vi "BTB Data Parser.vi"(8 "error in (no error)":errorcluster, 10 "RDS Serial Frame in":refnum<class "RDS Serial Frame.lvclass">, 11 "Battery Instrument in":refnum<class "Battery Instrument.lvclass">) -> (0 "error out":errorcluster, 2 "Battery Message out":refnum<class "Battery Message.lvclass">, 3 "Battery Instrument out":refnum<class "Battery Instrument.lvclass">)   [LabVIEW 2015, in "Battery Instrument.lvlib" / "Battery Instrument.lvclass"]
uses:
  Battery Instrument.lvclass
  Libraries/RDS Serial Handler/RDS Serial Frame.lvclass
  Libraries/RDS Child Messages/Battery Data/Battery Message.lvclass
  Libraries/RDS Serial Handler/RDS Serial Frame.lvclass/RDS Serial Frame.ctl
  Libraries/RDS Framework/RDS Message ID.ctl
  Libraries/RDS Instruments/Battery/Battery Data.ctl
  Libraries/RDS Child Messages/Battery Data/Battery Status.ctl
  Libraries/RDS Framework/RDS Message Class/RDS Message.lvclass/RDS Message.ctl
  Libraries/RDS Child Messages/Battery Data/Battery Message.lvclass/Battery Message.ctl
  Libraries/RDS Child Messages/RDS Child Messages.lvlib
  Libraries/RDS Framework/RDS Message Class/RDS Message.lvclass
  Libraries/RDS Serial Handler/RDS Serial Handler.lvlib
  Libraries/RDS Instruments/RDS Instrument Library.lvlib
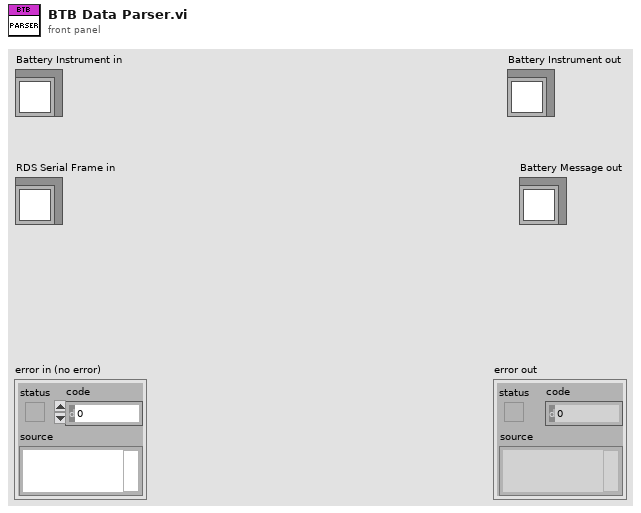
[diagram p1: front panel]
types:
  T1 = typedef "RDS Instrument Library.lvlib/Battery Data.ctl" = cluster{"Battery Status":T2, "Pack Voltage":sgl, "Pack Current":sgl, "Pack Capacity":sgl, "Max Cell Temp":sgl, "Min Cell Temp":sgl, "Max Cell Voltage":sgl, "Min Cell Voltage":sgl}
  T2 = typedef "RDS Instrument Library.lvlib/Battery Status.ctl" = enum16{"Pack Normal", "Alarm: Cell temp too high", "Alarm: Pack voltage too high", "Warn: Pack voltage too high ", "Alarm: Pack voltage too low", "Warn: Pack voltage low", "Alarm Pack current too high", "Warn: Pack current too high ", "Fault: Pack to chassis connection detected", "Fault: Pack to cell connection error", "Fautl: System error"}
  T3 = typedef "RDS Child Messages.lvlib/RDS Message ID.ctl" = enum16{"RDS Hello World", "String Message", "AIP_Status", "AIP_Command", "GPS_Data", "MCB_Command", "MCB_Status", "Compass_Data", "Depth_Data", "Battery_Data", "Contoller_State", "Set_Mag_Dev", "BTB_Shutdown", "State_Sample_Request", "State_Sample", "PID_Gains_Set", "Helm_Limiter_Set", "Helm_Heading_Command", "Helm_Steering_Command", "Helm_Status", "Controller_Message", "AIP_Set_Min_Depth", "Mission_Controller_State", "Mission_Upload", "Mission_Set_Op_and_Run", "Mission_Settings_Set"}
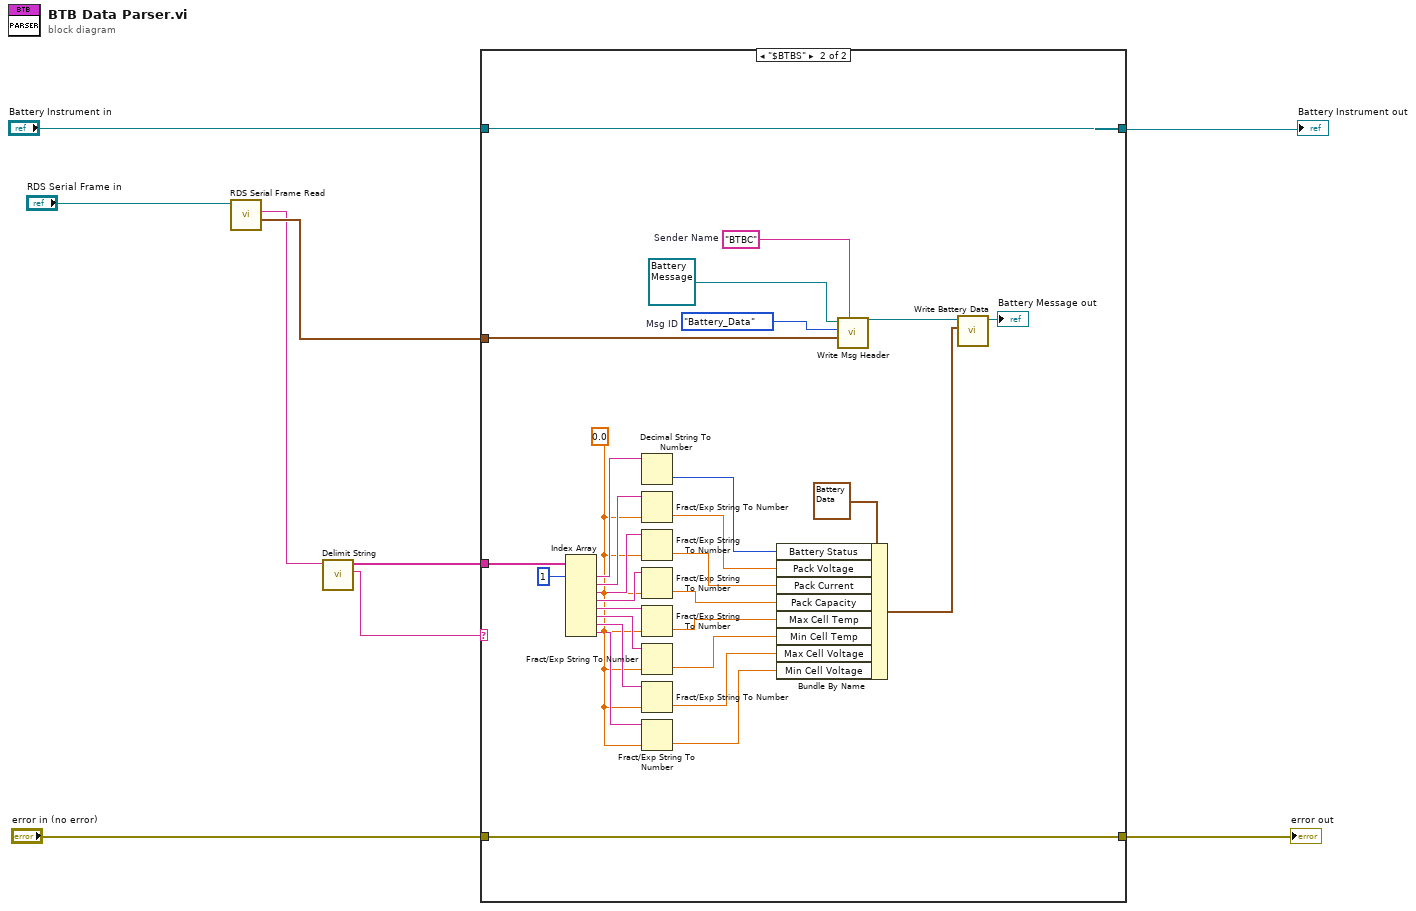
[diagram p0: block diagram]
diagram:
  n1 = call "RDS Serial Frame Read.vi"("RDS Serial Frame in"="RDS Serial Frame in") -> ("Time Stamp"=w7:timestamp, "Serial String"=w1:string)  [unwired: 7 in, 2 out]
  n2 = call "Delimit String.vi"("Serial String"=w1) -> ("First Element"=w8:string, "All Elements"=w9:string[])  [unwired: 9 in]
  n3 = case shown="\"$BTBS\"" w8 {
    tunnel: w9 -> [_ w40]
    tunnel: w7 -> [_ w38]
    tunnel: [w11 w35] -> w4
    tunnel: "Battery Instrument in" -> [w11 w35]
    tunnel: [w10 w34] -> w5
    tunnel: "error in (no error)" -> [w10 w34]
    frame "False", Default {
    }
    frame "$BTBS" {
      w12 = sgl 0.0 ("default (0 DBL)")
      w36 = "BTBC"  # Sender Name
      w37 = RDS_Message_ID."Battery_Data"  # Msg ID
      n4 = Index Array(array=w40, index #1=1 ("index")) -> (element #1=w29:string, element #2=w30:string, element #3=w26:string, element #4=w24:string, element #5=w22:string, element #6=w21:string, element #7=w20:string, element #8=w19:string)  [unwired: 7 in]
      n5 = Decimal String To Number(string=w29) -> (number=w28:i32)  [unwired: 2 in, 1 out]
      n6 = Fract/Exp String To Number(string=w30, default (0 dbl)=w12) -> (number=w27:sgl)  [unwired: 2 in, 1 out]
      n7 = Fract/Exp String To Number(string=w26, default (0 dbl)=w12) -> (number=w25:sgl)  [unwired: 2 in, 1 out]
      n8 = Fract/Exp String To Number(string=w24, default (0 dbl)=w12) -> (number=w23:sgl)  [unwired: 2 in, 1 out]
      n9 = Fract/Exp String To Number(string=w22, default (0 dbl)=w12) -> (number=w18:sgl)  [unwired: 2 in, 1 out]
      n10 = Fract/Exp String To Number(string=w21, default (0 dbl)=w12) -> (number=w17:sgl)  [unwired: 2 in, 1 out]
      n11 = Fract/Exp String To Number(string=w20, default (0 dbl)=w12) -> (number=w16:sgl)  [unwired: 2 in, 1 out]
      n12 = Fract/Exp String To Number(string=w19, default (0 dbl)=w12) -> (number=w15:sgl)  [unwired: 2 in, 1 out]
      n13 = Bundle By Name(cluster=T1 {"Battery Status"=enum."Pack Normal", "Pack Voltage"=0.0, "Pack Current"=0.0, "Pack Capacity"=0.0, "Max Cell Temp"=0.0, "Min Cell Temp"=0.0, "Max Cell Voltage"=0.0, "Min Cell Voltage"=0.0} ("Battery Pack Info"), "Battery Status"=w28, "Pack Voltage"=w27, "Pack Current"=w25, "Pack Capacity"=w23, "Max Cell Temp"=w18, "Min Cell Temp"=w17, "Max Cell Voltage"=w16, "Min Cell Voltage"=w15) -> (w14:T1)
      n14 = call "Write Msg Header.vi"("Sender Name"=w36, "Time Stamp"=w38, "Msg ID"=w37, "RDS Message in"=refnum<class "Battery Message.lvclass"> refnum ("RDS Child Messages.lvlib:Battery Message.lvclass")) -> ("RDS Message out"=w32:refnum<class "Battery Message.lvclass">)  [unwired: 6 in, 1 out]
      n15 = call "Write Battery Data.vi"("Battery Pack Info"=w14, "Battery Message in"=w32) -> ("Battery Message out"=→"Battery Message out":refnum<class "Battery Message.lvclass">)  [unwired: 8 in, 1 out]
    }
  }
  "error out" <- w5
  "Battery Instrument out" <- w4
